vi "Agilent MXA Series Acquire Measurement.vi"() -> ()   [LabVIEW 2018]
doc: "This example shows how to configure the spectrum analyzer to acquire measurement."
uses:
  Public/Configure/Configure Frequency (Start Stop).vi
  Public/Configure/Configure Level (Normal).vi
  Public/Configure/Measurement/Configure Measurement (Channel Power).vi
  Public/Data/Read Measurement (Channel Power Measurement).vi
  Agilent MXA Series.lvlib
panel:
  in  "Mechanical Attenuation Step (0: 2 dB)":i32(ring) items=["2", "10"]
  in  "Manual Mechanical Attenuation (10 dB)":dbl=10.0
  out "Power Spectral Density":dbl
  out "Channel Power":dbl
  in  "Filter Bandwidth (3.84 E+6 Hz)":dbl=3840000.0
  in  "Filter Alpha (0.22)":dbl=0.22 format="%#.6g"
  in  "Averaging Mode (0: Exponential)":i32(ring) items=["Exponential", "Repeat"]
  in  "Average Number (10)":i32=10 format="%.0g"
  in  "Timeout (50000 ms)":i32=50000 format="%.0g"
  in  "Reference Level Offset (0 dB)":dbl
  in  "Reference Level (10 dBm)":dbl=10.0
  in  "Input Impedance (0: 50 ohms)":i32(ring) items=["50", "75"]
  in  "Stop Frequency (25 E+9 Hz)":dbl=25000000000.0
  in  "Start Frequency (100 E+3 Hz)":dbl=100000.0
  in  "VISA resource name":refnum<visa-resource-name>
  # "(c) 2007-2015 National Instruments.  ALL RIGHTS RESERVED."
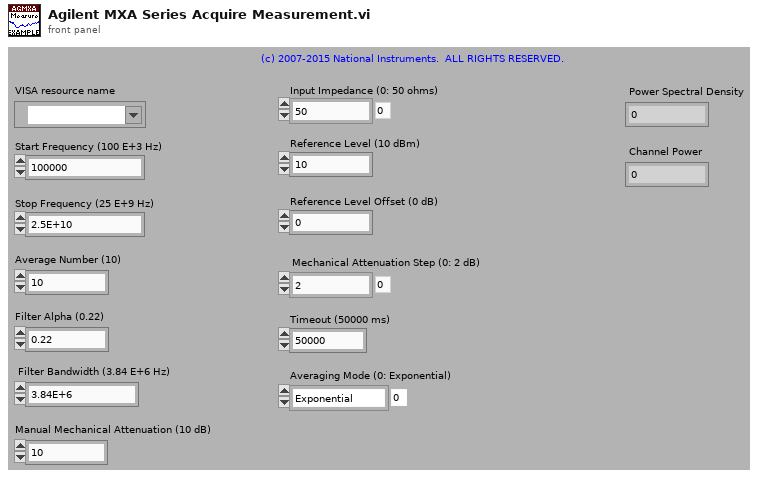
[diagram p1: front panel]
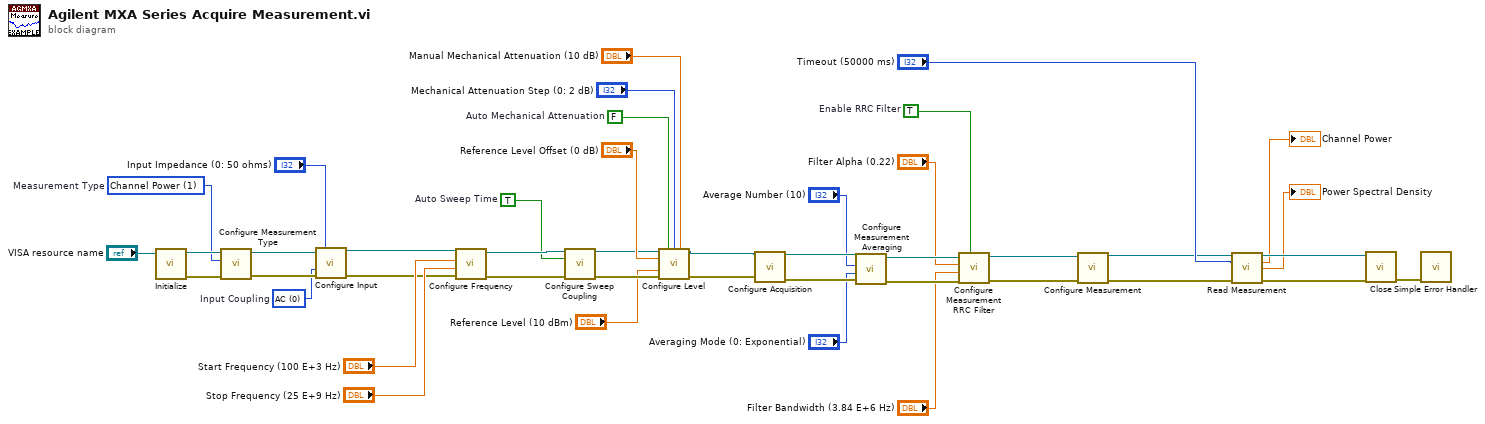
[diagram p0: block diagram]
diagram:
  w3 = FALSE  # Auto Mechanical Attenuation
  w4 = TRUE  # Enable RRC Filter
  w31 = 0 items=["AC", "DC"]  # Input Coupling
  w35 = 1 items=["Swept SA", "Channel Power", "Occupied Bandwidth", "Power Stat CCDF", "Adjacent Channel Power", "Burst Power", "Spurious Emissions", "Spectrum Emission Mask", "List Sweep"]  # Measurement Type
  w34 = TRUE  # Auto Sweep Time
  n1 = call "Initialize.vi"("VISA resource name"="VISA resource name") -> ("error out"=w38:errorcluster, "VISA resource name out"=w39:refnum<visa-resource-name>)  [unwired: 9 in]
  n2 = call "Configure Measurement Type.vi"("error in (no error)"=w38, "Measurement Type (0: Swept SA)"=w35, "VISA resource name"=w39) -> ("error out"=w32:errorcluster, "VISA resource name out"=w33:refnum<visa-resource-name>)  [unwired: 7 in]
  n3 = call "Configure Input.vi"("VISA resource name"=w33, "Input Impedance (0: 50 ohms)"="Input Impedance (0: 50 ohms)", "Input Coupling  (0: AC)"=w31, "error in (no error)"=w32) -> ("VISA resource name out"=w23:refnum<visa-resource-name>, "error out"=w22:errorcluster)  [unwired: 10 in]
  n4 = call-poly "Configure Frequency.vi"("error in (no error)"=w22, "Stop Frequency (2.65E+10 Hz)"="Stop Frequency (25 E+9 Hz)", "Start Frequency (1E+7 Hz)"="Start Frequency (100 E+3 Hz)", "VISA resource name"=w23) -> ("error out"=w36:errorcluster, "VISA resource name out"=w37:refnum<visa-resource-name>)  [unwired: 6 in]
  n5 = call "Configure Sweep Coupling.vi"("VISA resource name"=w37, "Auto Sweep Time (T: Enable)"=w34, "error in (no error)"=w36) -> ("VISA resource name out"=w24:refnum<visa-resource-name>, "error out"=w29:errorcluster)  [unwired: 11 in]
  n6 = call-poly "Configure Level.vi"("VISA resource name"=w24, "Auto Mechanical Attenuation (T: Enable)"=w3, "Mechanical Attenuation Step (0: 2 dB)"="Mechanical Attenuation Step (0: 2 dB)", "Manual Mechanical Attenuation (10 dB)"="Manual Mechanical Attenuation (10 dB)", "Reference Level (0 dBm)"="Reference Level Offset (0 dB)", "Amplitude Units (0: dBm)"="Reference Level (10 dBm)", "error in (no error)"=w29) -> ("VISA resource name out"=w27:refnum<visa-resource-name>, "error out"=w28:errorcluster)  [unwired: 7 in]
  n7 = call "Configure Acquisition.vi"("VISA resource name"=w27, "error in (no error)"=w28) -> ("VISA resource name out"=w21:refnum<visa-resource-name>, "error out"=w20:errorcluster)  [unwired: 12 in]
  n8 = call "Configure Measurement Averaging.vi"("error in (no error)"=w20, "Averaging Mode (0: Exponential)"="Averaging Mode (0: Exponential)", "Average Number (10)"="Average Number (10)", "VISA resource name"=w21) -> ("error out"=w16:errorcluster, "VISA resource name out"=w17:refnum<visa-resource-name>)  [unwired: 6 in]
  n9 = call "Configure Measurement RRC Filter.vi"("Enable RRC Filter (F: Disable)"=w4, "error in (no error)"=w16, "Filter Bandwidth (3.84E+6 Hz)"="Filter Bandwidth (3.84 E+6 Hz)", "Filter Alpha (0.22)"="Filter Alpha (0.22)", "VISA resource name"=w17) -> ("error out"=w15:errorcluster, "VISA resource name out"=w14:refnum<visa-resource-name>)  [unwired: 5 in]
  n10 = call-poly "Configure Measurement.vi"("VISA resource name"=w14, "error in (no error)"=w15) -> ("VISA resource name out"=w10:refnum<visa-resource-name>, "error out"=w9:errorcluster)  [unwired: 12 in]
  n11 = call-poly "Read Measurement.vi"("VISA resource name"=w10, "Timeout (10000 ms)"="Timeout (50000 ms)", "error in (no error)"=w9) -> ("VISA resource name out"=w8:refnum<visa-resource-name>, "Channel Power"=→"Channel Power":dbl, "Power Spectral Density"=→"Power Spectral Density":dbl, "error out"=w7:errorcluster)  [unwired: 9 in]
  n12 = call "Close.vi"("error in (no error)"=w7, "VISA resource name"=w8) -> ("error out"=w43:errorcluster)  [unwired: 9 in]
  n13 = call <vilib>:"Simple Error Handler.vi"("error in (no error)"=w43) -> ()  [unwired: 4 in, 5 out]
